vi "VS-Read Temp (general).vi"(8 "error in (no error)":errorcluster, 11 "Scale":T1={"Slope"=0.0, "Offset"=0.0, "Limits"={"Min"=0.0, "Max"=0.0}, "term config"=-1} {"term config" items=["default"=-1, "RSE"=10083, "NRSE"=10078, "Differential"=10106, "Pseudodifferential"=12529]}) -> (0 "error out":errorcluster, 2 "Vmean":dbl, 3 "Temp (C)":dbl)   [LabVIEW 2020]
uses:
  Typedefs/PhysMon-Scale.ctl
  epl-vi-lib/Connection VIs/Type Defs/Input sources.ctl
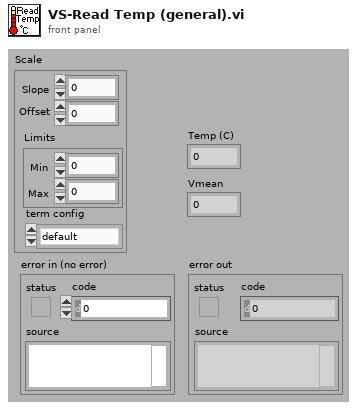
[diagram p1: front panel]
types:
  T1 = typedef "PhysMon-Scale.ctl" = cluster{"Slope":dbl, "Offset":dbl, "Limits":cluster{"Min":dbl, "Max":dbl}, "term config":i32}
  T2 = typedef "Input sources.ctl" = u16
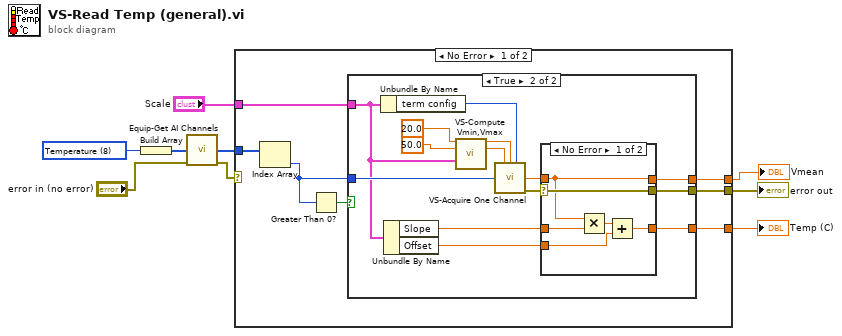
[diagram p0: block diagram]
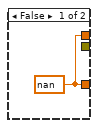
[diagram p2: hidden frame]
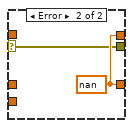
[diagram p3: hidden frame]
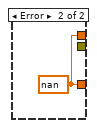
[diagram p4: hidden frame]
diagram:
  w9 = T2 8 items=["--unused--", "Probe Mic Right", "Probe Mic Left", "Cal Mic", "ABR", "CAP Right", "CAP Left", "Startle piezo", "Temperature", "Heart rate"] ("Ring")
  n1 = Build Array(w9) -> (w8:T2[])
  n2 = call "Equip-Get AI Channels.vi"("Inputs"=w8, "error in (no error)"="error in (no error)") -> ("AI Channels"=w7:i32[], "error out"=w6:errorcluster)  [unwired: 12 in]
  n3 = case shown="No Error" w6 {
    tunnel: [w16 w40] -> w5
    tunnel: w7 -> [w15 _]
    tunnel: "Scale" -> [w12 _]
    tunnel: [w11 _] -> w2
    tunnel: [w10 w40] -> w1
    frame No Error {
      n4 = Index Array(array=w15) -> (element=w14:i32)  [unwired: 1 in]
      n5 = Greater Than 0?(x=w14) -> (x > 0?=w13:bool)
      n6 = case shown="True" w13 {
        tunnel: [w17 w28] -> w16
        tunnel: w14 -> [_ w30]
        tunnel: w12 -> [_ w24]
        tunnel: [_ w25] -> w11
        tunnel: [w17 w19] -> w10
        frame False {
          w17 = nan
        }
        frame True {
          n7 = Unbundle By Name(w24) -> ("term config"=w18:i32)
          n8 = Unbundle By Name(w24) -> ("Slope"=w29:dbl, "Offset"=w27:dbl)
          n9 = call "VS-Compute Vmin,Vmax.vi"("Min"=20.0, "Max"=50.0, "Scale"=w24) -> ("Vmin"=w23:dbl, "Vmax"=w22:dbl)  [unwired: 10 in, 1 out]
          n10 = call "VS-Acquire One Channel.vi"("maximum value"=w22, "minimum value"=w23, "input terminal configuration"=w18, "index"=w30) -> ("mean"=w31:dbl, "error out"=w26:errorcluster)  [unwired: 10 in]
          n11 = case shown="No Error" w26 {
            selector: w26 -> [w33 w38]
            tunnel: w31 -> [w32 _]
            tunnel: w29 -> [w36 _]
            tunnel: [w35 w39] -> w28
            tunnel: w27 -> [w34 _]
            tunnel: [w33 w38] -> w25
            tunnel: [w32 w39] -> w19
            frame No Error {
              n12 = Multiply(x=w32, y=w36) -> (x*y=w37:dbl)
              n13 = Add(x=w37, y=w34) -> (x+y=w35:dbl)
            }
            frame Error {
              w39 = nan
            }
          }
        }
      }
    }
    frame Error {
      w40 = nan
    }
  }
  "error out" <- w2
  "Temp (C)" <- w5
  "Vmean" <- w1
